vi "Configure Source.vi"(8 "error in (no error)":errorcluster, 10 "Source (F:Volt)":bool, 11 "Keithley 24xx in":refnum<class "Keithley 24xx.lvclass">) -> (0 "error out":errorcluster, 3 "Keithley 24xx out":refnum<class "Keithley 24xx.lvclass">)   [LabVIEW 2020, in "Keithley 24xx.lvclass"]
uses:
  Keithley 24xx.lvclass
  C:/Sandbox/Git_Sandbox/WiSpry Test Framework source code (LV20)/WiSpry Test Framework/Instruments/Instrument.lvclass
  C:/Sandbox/Git_Sandbox/WiSpry Test Framework source code (LV20)/WiSpry Test Framework/Instruments/Power Supply/Power Supply.lvclass
  Instrument.lvclass/Instrument.ctl
  Instrument.lvclass
  <instrlib>/Keithley 24XX/Keithley 24XX.lvlib
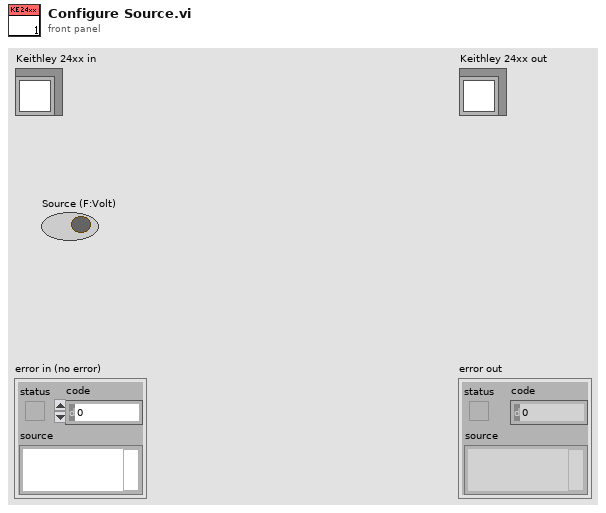
[diagram p1: front panel]
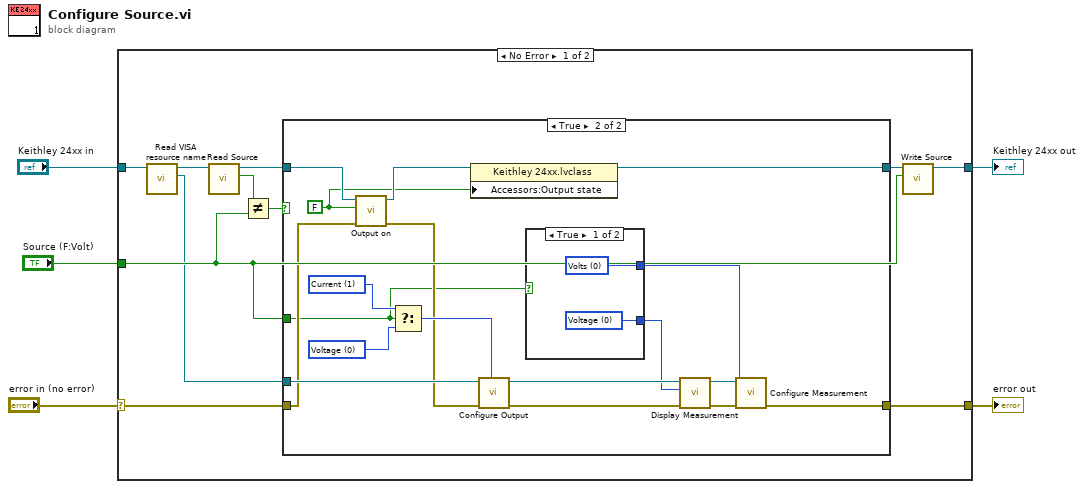
[diagram p0: block diagram]
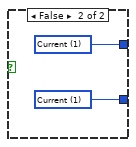
[diagram p3: hidden frame]
diagram:
  n1 = case shown="No Error" "error in (no error)" {
    selector: "error in (no error)" -> [w11 w42]
    tunnel: [w8 w42] -> w4
    tunnel: [w15 w41] -> w3
    tunnel: "Keithley 24xx in" -> [w16 w41]
    tunnel: "Source (F:Volt)" -> [w10 _]
    frame No Error {
      n2 = call "Read VISA resource name.vi"("Instrument in"=w16) -> ("VISA resource name"=w9:refnum<visa-resource-name>, "Instrument out"=w14:refnum<class "Keithley 24xx.lvclass">)  [unwired: 9 in]
      n3 = call-dynamic "Read Source.vi"("Power Supply in"=w14) -> ("Source"=w13:bool, "Power Supply out"=w7:refnum<class "Keithley 24xx.lvclass">)  [unwired: 9 in]
      n4 = Not Equal?(x=w13, y=w10) -> (x != y?=w12:bool)
      n5 = case shown="True" w12 {
        tunnel: w11 -> [w18 w29]
        tunnel: w10 -> [_ w19]
        tunnel: w9 -> [_ w33]
        tunnel: [w18 w22] -> w8
        tunnel: w7 -> [w17 w32]
        tunnel: [w17 w28] -> w6
        frame False {
        }
        frame True {
          w27 = FALSE ("Output On")
          w36 = u16 1 items=["Voltage", "Current"] ("Source Mode  (0: Voltage)")
          w35 = u16 0 items=["Voltage", "Current"] ("Source Mode  (0: Voltage)")
          n6 = call-dynamic "Output on.vi"("error in (no error)"=w29, "Output On"=w27, "Keithley 24xx in"=w32) -> ("error out"=w30:errorcluster, "Keithley 24xx out"=w31:refnum<class "Keithley 24xx.lvclass">)  [unwired: 7 in]
          n7 = Select(t=w36, s=w19, f=w35) -> (s? t:f=w34:u16)
          n8 = property class="Keithley 24xx.lvclass"(reference=w31, "Accessors:Output state"=w27) -> (reference out=w28:refnum<class "Keithley 24xx.lvclass">)  [unwired: 1 in, 1 out]
          n9 = call <instrlib>:"Configure Output.vi"("Source Mode  (0: Voltage)"=w34, "error in (no error)"=w30, "VISA resource name"=w33) -> ("error out"=w23:errorcluster, "VISA resource name out"=w24:refnum<visa-resource-name>)  [unwired: 7 in]
          n10 = case shown="True" w19 {
            tunnel: [w38 w40] -> w21
            tunnel: [w37 w39] -> w20
            frame True {
              w37 = u16 0 items=["Voltage", "Current", "Resistance"] ("Displayed Measurement (0: Voltage)")
              w38 = u16 0 items=["Volts", "Current", "Resistance"] ("Function (0: Volts)")
            }
            frame False {
              w39 = u16 1 items=["Voltage", "Current", "Resistance"] ("Displayed Measurement (0: Voltage)")
              w40 = u16 1 items=["Volts", "Current", "Resistance"] ("Function (0: Volts)")
            }
          }
          n11 = call <instrlib>:"Display Measurement.vi"("error in (no error)"=w23, "Displayed Measurement (0: Voltage)"=w20, "VISA resource name"=w24) -> ("error out"=w25:errorcluster, "VISA resource name out"=w26:refnum<visa-resource-name>)  [unwired: 7 in]
          n12 = call <instrlib>:"Configure Measurement.vi"("error in (no error)"=w25, "Function (0: Volts)"=w21, "VISA resource name"=w26) -> ("error out"=w22:errorcluster)  [unwired: 7 in, 1 out]
        }
      }
      n13 = call-dynamic "Write Source.vi"("Source"=w10, "Power Supply in"=w6) -> ("Power Supply out"=w15:refnum<class "Keithley 24xx.lvclass">)  [unwired: 9 in]
    }
    frame Error {
    }
  }
  "error out" <- w4
  "Keithley 24xx out" <- w3
